vi "synnax writer open.vi"(4 "enable_auto_commit (T)":bool=TRUE, 5 "err_on_unauthorized (F)":bool, 6 "auto_index (F)":bool, 7 "start (now)":timestamp, 8 "error in":errorcluster, 9 "authorities (255 for all channels)":u8[](array[numeric]), 10 "channels":u32[](array[numeric]), 11 "client in":u64) -> (0 "error out":errorcluster, 3 "writer out":u64)   [LabVIEW 2026, in "synnax_clib.lvlib"]
doc: "SYNNAX_EXPORT int32_t synnax_writer_open(\n SynnaxClient client,\n int64_t start,\n const uint32_t *channels,\n uint64_t channel_count,\n int32_t mode,\n int32_t enable_auto_commit,\n SynnaxWriter *out_writer,\n SynnaxError err\n);"
uses:
  synnax_clib.lvlib
  typedefs/writer_mode.ctl
  synnax_clib.dll
panel:
  out "client out":u64
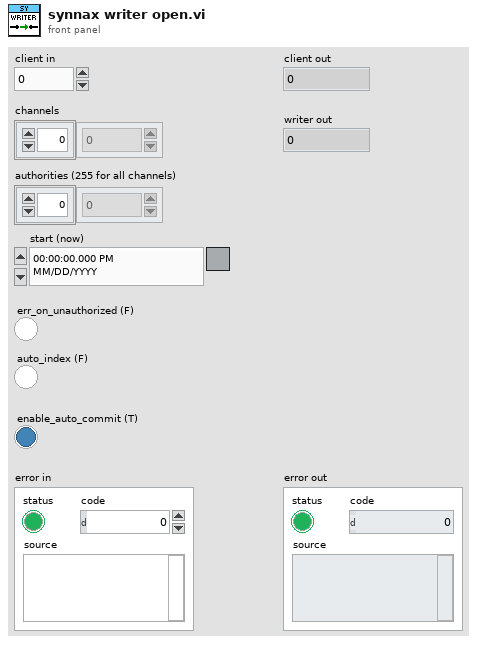
[diagram p1: front panel]
types:
  T1 = typedef "synnax_clib.lvlib/writer_mode.ctl" = enum16{"PERSIST & STREAM", "PERSIST", "STREAM"}
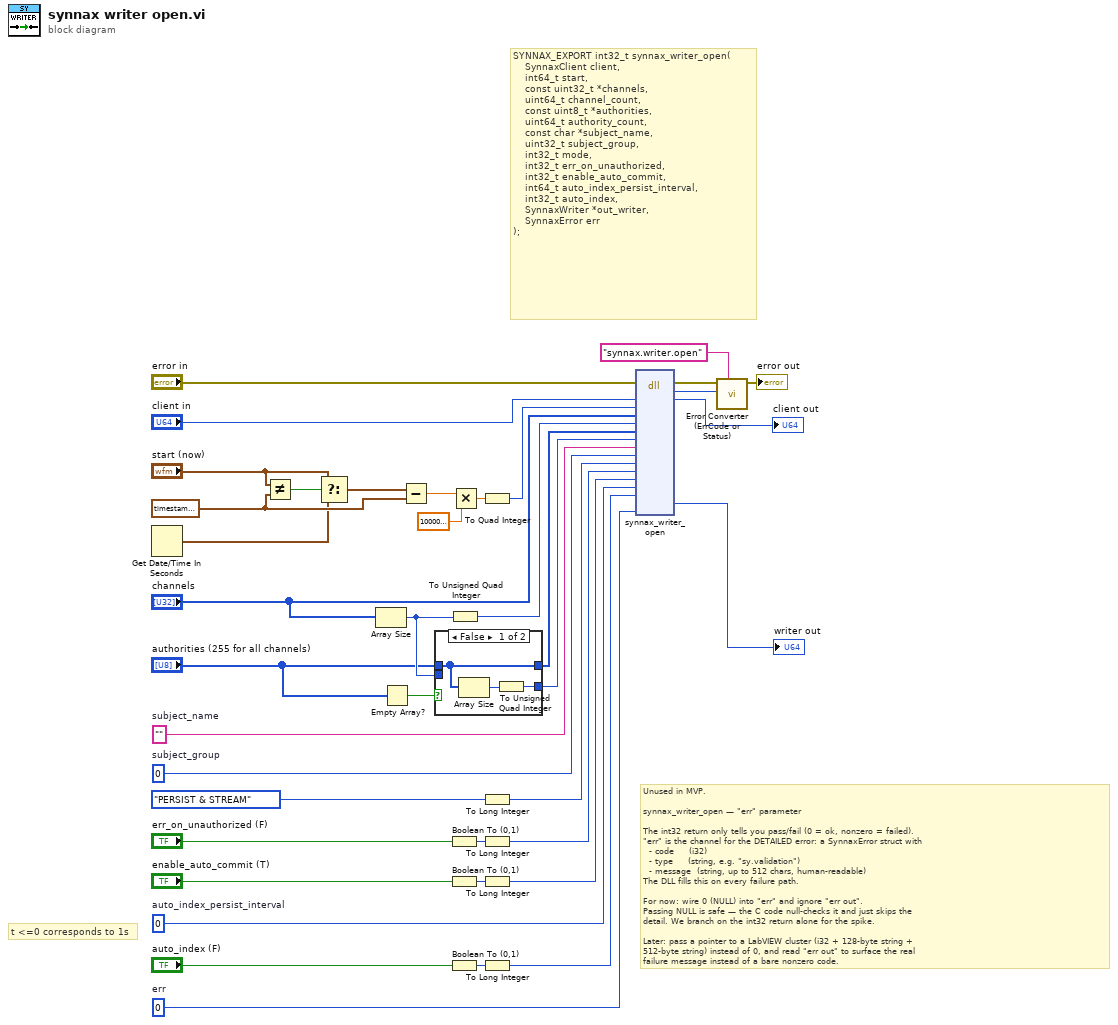
[diagram p0: block diagram]
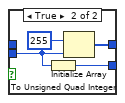
[diagram p2: hidden frame]
diagram:
  w3 = timestamp timestamp(0 s since 1904-01-01)
  w15 = i64 0  # auto_index_persist_interval
  w19 = u32 0  # subject_group
  w20 = ""  # subject_name
  w34 = u64 0  # err
  # "t <=0 corresponds to 1s"
  # "Unused in MVP.\n\nsynnax_writer_open — \"err\" parameter\n\nThe int32 return only tells you pass/fail (0 = ok, nonzero = failed).\n\"err\" is the channel for the DETAILED error: a SynnaxError struct with\n  - code     (i32)\n  - type     (string, e.g. \"sy.validation\")\n  - message  (string, up to 512 chars, human-readable)\nThe DLL fills this on every failure path.\n\nFor now: wire 0 (NULL) into \"err\" and ignore \"err out\".\nPassing NULL is safe — the C code null-checks it and just skips the\ndetail. We branch on the int32 return alone for the spike.\n\nLater: pass a pointer to a LabVIEW cluster (i32 + 128-byte string +\n512-byte string) instead of 0, and read \"err out\" to surface the real\nfailure message instead of a bare nonzero code."
  # "SYNNAX_EXPORT int32_t synnax_writer_open(\n    SynnaxClient client,\n    int64_t start,\n    const uint32_t *channels,\n    uint64_t channel_count,\n    const uint8_t *authorities,\n    uint64_t authority_count,\n    const char *subject_name,\n    uint32_t subject_group,\n    int32_t mode,\n    int32_t err_on_unauthorized,\n    int32_t enable_auto_commit,\n    int64_t auto_index_persist_interval,\n    int32_t auto_index,\n    SynnaxWriter *out_writer,\n    SynnaxError err\n);"
  n1 = Get Date/Time In Seconds() -> (seconds since 1Jan1904=w1:timestamp)
  n2 = Not Equal?(x="start (now)", y=w3) -> (x != y?=w5:bool)
  n3 = Select(t="start (now)", s=w5, f=w1) -> (s? t:f=w4:timestamp)
  n4 = Array Size(array="channels") -> (size(s)=w10:i32)
  n5 = Empty Array?(array="authorities (255 for all channels)") -> (empty?=w8:bool)
  n6 = Subtract(x=w4, y=w3) -> (x-y=w33:dbl)
  n7 = case shown="False" w8 {
    tunnel: [w41 w46] -> w11
    tunnel: w10 -> [_ w44]
    tunnel: "authorities (255 for all channels)" -> [w41 _]
    tunnel: [w40 w43] -> w6
    frame False {
      n8 = Array Size(array=w41) -> (size(s)=w42:i32)
      n9 = To Unsigned Quad Integer(1:w42) -> (0:w40:u64)
    }
    frame True {
      n10 = To Unsigned Quad Integer(1:w44) -> (0:w43:u64)
      n11 = Initialize Array(u8 255, w44) -> (w46:u8[])
    }
  }
  n12 = Boolean To (0,1)(Boolean="err_on_unauthorized (F)") -> (0, 1=w17:i16)
  n13 = Boolean To (0,1)(Boolean="enable_auto_commit (T)") -> (0, 1=w35:i16)
  n14 = Boolean To (0,1)(Boolean="auto_index (F)") -> (0, 1=w13:i16)
  n15 = To Unsigned Quad Integer(1:w10) -> (0:w9:u64)
  n16 = Multiply(x=w33, y=1000000000.0) -> (x*y=w31:dbl)
  n17 = To Quad Integer(1:w31) -> (0:w30:i64)
  n18 = To Long Integer(number=writer_mode."PERSIST & STREAM") -> (32bit integer=w21:i32)
  n19 = To Long Integer(number=w17) -> (32bit integer=w16:i32)
  n20 = To Long Integer(number=w35) -> (32bit integer=w29:i32)
  n21 = To Long Integer(number=w13) -> (32bit integer=w12:i32)
  n22 = dll-call lib="C/synnax/client/labview/synnax_clib.*" fn="synnax_writer_open"(error in="error in", "client"="client in", "start"=w30, "channels"="channels", "channel_count"=w9, "authorities"=w11, "authority_count"=w6, "subject_name"=w20, "subject_group"=w19, "mode"=w21, "err_on_unauthorized"=w16, "enable_auto_commit"=w29, "auto_index_persist_interval"=w15, "auto_index"=w12, "err"=w34) -> (error out=w28:errorcluster, "return type"=w27:i32, "client"=→"client out":u64, "out_writer"=→"writer out":u64)  [unwired: 16 in, 1 out]
  n23 = call "Error Converter (ErrCode or Status).vi"("source"="synnax.writer.open", "error code"=w27, "error in (no error)"=w28) -> ("error out"=→"error out":errorcluster)  [unwired: 8 in]
